vi "Component_Init.vi"(8 "Error In":errorcluster, 10 "WebView2":refnum<k24>(container), 11 "object in":refnum<class "Component.lvclass">) -> (0 "Error Out":errorcluster, 3 "object out":refnum<class "Component.lvclass">)   [LabVIEW 2020, in "Component.lvclass"]
uses:
  Component.lvclass
  Component.lvclass/Component.ctl
  <vilib>/sklein/WebView2/Webview2 Lib/WebView2 Control Object/WebView2 Control.lvclass
  <vilib>/sklein/WebView2/Libs/Microsoft.Web.WebView2.WinForms.dll
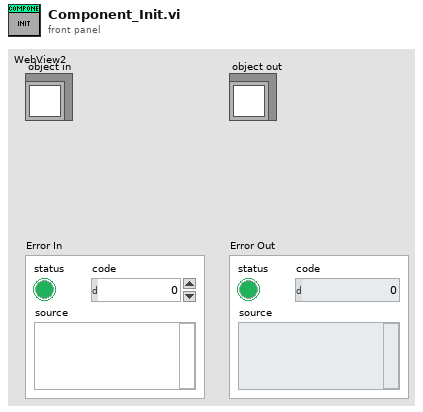
[diagram p1: front panel]
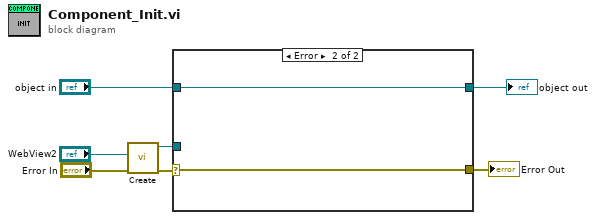
[diagram p0: block diagram]
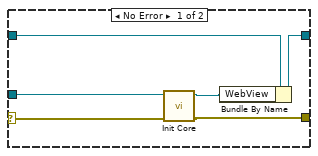
[diagram p2: hidden frame]
diagram:
  n1 = call <vilib>:"Create.vi"("error in (no error)"="Error In", "WebView2 Control"="WebView2") -> ("error out"=w3:errorcluster, "WebView2 Control out"=w4:refnum<class "WebView2 Control.lvclass">)  [unwired: 8 in]
  n2 = case shown="Error" w3 {
    selector: w3 -> [w10 w14]
    tunnel: "object in" -> [w13 w15]
    tunnel: [w12 w15] -> w6
    tunnel: w4 -> [w11 _]
    tunnel: [w9 w14] -> w1
    frame No Error {
      n3 = call <vilib>:"Init Core.vi"("error in (no error)"=w10, "WebView2 Control in"=w11) -> ("error out"=w9:errorcluster, "WebView2 Control out"=w8:refnum<class "WebView2 Control.lvclass">)  [unwired: 8 in]
      n4 = Bundle By Name(cluster=w13, "WebView"=w8) -> (w12:refnum<class "Component.lvclass">)
    }
    frame Error {
    }
  }
  "object out" <- w6
  "Error Out" <- w1
